vi "Update UI.vi"(8 "error in (no error)":errorcluster, 10 "DataExchange":T1, 11 "Controller Template in":refnum<class "QuickNoteUI.lvclass">) -> (0 "error out":errorcluster, 3 "Controller Template out":refnum<class "QuickNoteUI.lvclass">)   [LabVIEW 2020]
uses:
  QuickNoteUI.lvclass
  E:/Development/DevHardSoftware/MicroscopyFramework/Model/Hardware Abstraction Layer/Component/GenericActor/GenericActor/GenericController.lvclass
  C:/Program Files/National Instruments/LabVIEW 2020/vi.lib/ActorFramework/Actor/Actor.lvclass
  E:/Development/DevHardSoftware/MicroscopyFramework/Interface/DataGenerator/DataGenerator.lvclass
  E:/Development/DevHardSoftware/MicroscopyFramework/Interface/DataListener/DataListener.lvclass
  E:/Development/DevHardSoftware/MicroscopyFramework/Interface/ErrorHandler/ErrorHandler.lvclass
  E:/Development/DevHardSoftware/MicroscopyFramework/Model/Logic Layer/QuickNoteUI/QuickNoteUI.lvclass
  Hardware Abstraction Layer/Component/Device/Device/DataExchange.ctl
  Interface/DataListener/DataListener.lvclass
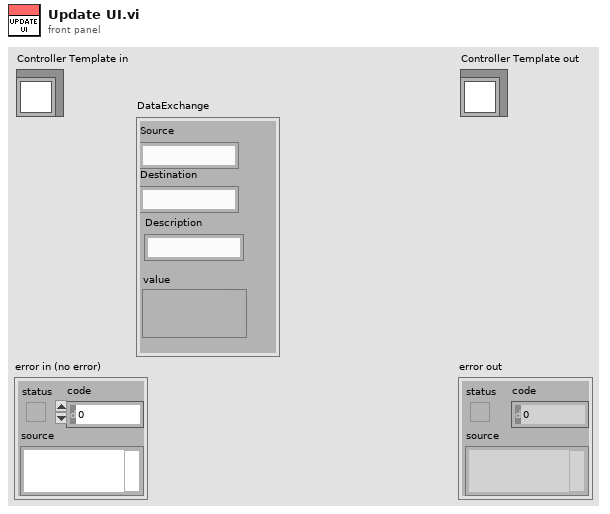
[diagram p1: front panel]
types:
  T1 = typedef "DataListener.lvclass/DataExchange.ctl" = cluster{"Source":string, "Destination":string, "Description":string, "value":variant}
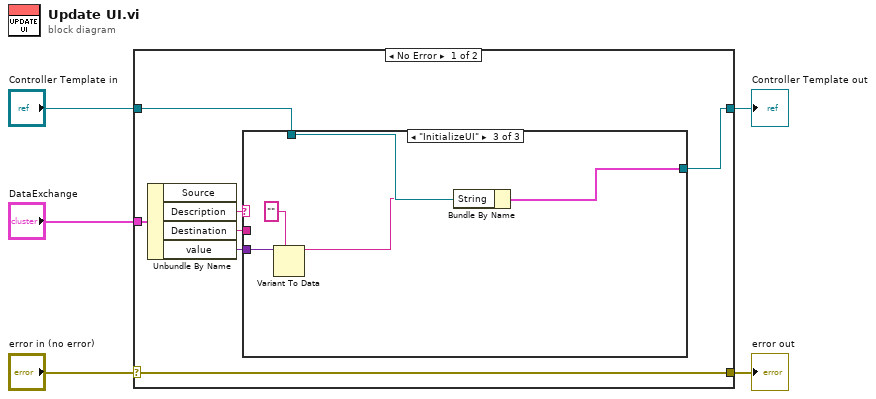
[diagram p0: block diagram]
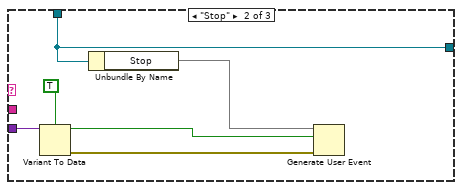
[diagram p3: hidden frame]
diagram:
  n1 = case shown="No Error" "error in (no error)" {
    selector: "error in (no error)" -> [w12 w26]
    tunnel: [w12 w26] -> w4
    tunnel: [w6 w25] -> w2
    tunnel: "Controller Template in" -> [w7 w25]
    tunnel: "DataExchange" -> [w11 _]
    frame No Error {
      n2 = Unbundle By Name(w11) -> ("Description"=w8:string, "Destination"=w9:string, "value"=w10:variant)  [unwired: 1 out]
      n3 = case shown="\"InitializeUI\"" w8 {
        tunnel: w10 -> [_ w19 w24]
        tunnel: w9 -> [_ _ _]
        tunnel: w7 -> [w13 w14 w23]
        tunnel: [w13 w14 w22] -> w6
        frame Default {
        }
        frame "Stop" {
          n4 = Variant To Data(type=TRUE, Variant=w19) -> (data=w17:bool, error out=w15:errorcluster)  [unwired: 1 in]
          n5 = Unbundle By Name(w14) -> ("Stop"=w18)
          n6 = Generate User Event(user event=w18, event data cluster=w17, error in=w15) -> ()  [unwired: 1 in, 2 out]
        }
        frame "InitializeUI" {
          n7 = Variant To Data(type="" ("String"), Variant=w24) -> (data=w20:string)  [unwired: 1 in, 1 out]
          n8 = Bundle By Name(cluster=w23, "String"=w20) -> (w22:cluster{})
        }
      }
    }
    frame Error {
    }
  }
  "error out" <- w4
  "Controller Template out" <- w2
